vi "Initialise Motion.vi"(4 "Initial Velocity [m/s]":sgl=1.0 format="%#_13g", 5 "Field Size":T1={"x"=500.0, "y"=500.0}, 6 "Initial Heading [deg]":sgl=45.0 format="%#_13g", 7 "Maximum Velocity [m/s]":sgl=10.0 format="%.3g", 8 "Initial Position":T1, 9 "Acceleration [m/s/s]":sgl=10.0 format="%.3g", 10 "Turn Rate [deg/s]":sgl=90.0 format="%.3g", 11 "Element in":refnum<class "Element.lvclass">) -> (3 "Element out":refnum<class "Element.lvclass">)   [LabVIEW 2021, in "Element.lvclass"]
uses:
  Element.lvclass
  Element.lvclass/Element.ctl
  Motion/Motion.lvclass
  Math/Vec2.ctl
  Math/Math.lvlib
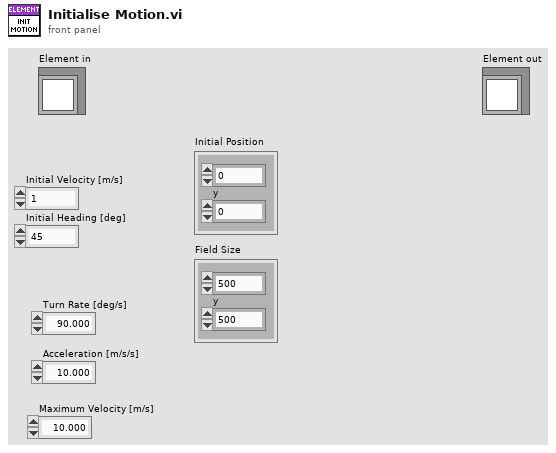
[diagram p1: front panel]
types:
  T1 = typedef "Math.lvlib/Vec2.ctl" = cluster{"x":sgl, "y":sgl}
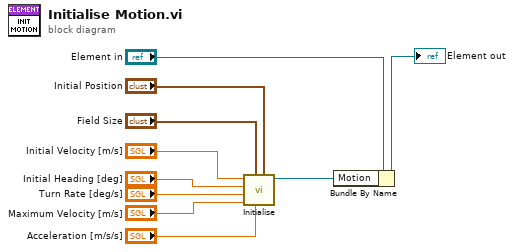
[diagram p0: block diagram]
diagram:
  n1 = call "Initialise.vi"("Initial Position"="Initial Position", "Acceleration [m/s/s]"="Acceleration [m/s/s]", "Field Size"="Field Size", "Maximum Velocity [m/s]"="Maximum Velocity [m/s]", "Turn Rate [deg/s]"="Turn Rate [deg/s]", "Initial Heading [deg]"="Initial Heading [deg]", "Initial Velocity [m/s]"="Initial Velocity [m/s]") -> ("Motion out"=w9:refnum<class "Motion.lvclass">)  [unwired: 4 in]
  n2 = Bundle By Name(cluster="Element in", "Motion"=w9) -> (→"Element out":refnum<class "Element.lvclass">)
